vi "Useful Values.vi"() -> ()   [LabVIEW 2013]
uses:
  <vilib>/Rock Robotics/WPI/DriverStation/WPI_DriverStationAllianceInfo.ctl
panel:
  in  "Percent Speed":dbl=0.4
  in  "SLOW?":bool=TRUE
  in  "Climbing":bool
  in  "Climbed":bool
  in  "Shooting":bool
  out "Alliance":T1
  in  "Homing Speed":dbl
  in  "Homing?":bool
  in  "Auto RPM":dbl
  in  "Gyro Turn":dbl
  in  "Shooter on":bool
  in  "Elevator Position Auto":dbl=2.5
  in  "Motor Speed":dbl
  in  "Spun up?":bool
  in  "Competition":bool
  in  "RPM Wanted":dbl=1812.0
  in  "Auto?":bool
  in  "Correcting?":bool
  out "Current RPM":dbl
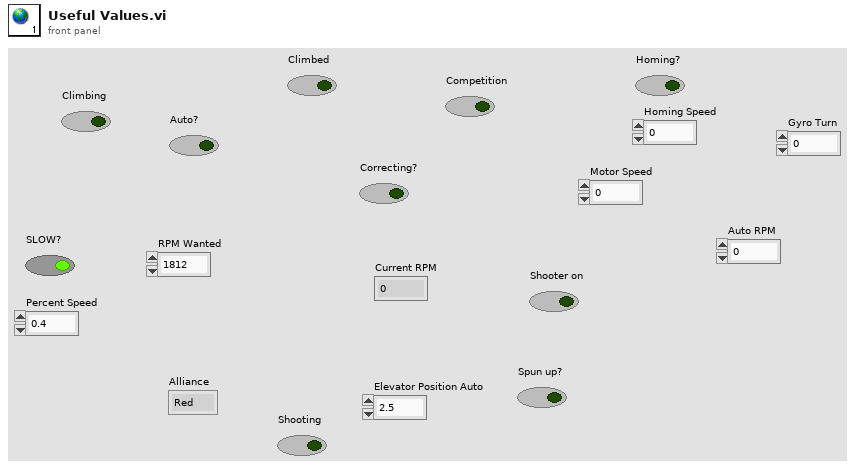
[diagram p1: front panel]
types:
  T1 = typedef "WPI_DriverStationAllianceInfo.ctl" = enum16{"Red", "Blue", "Invalid"}
diagram:
